vi "Read SecretKey.vi"(8 "error in (no error)":errorcluster, 11 "Attribute.Identity in":refnum<class "Attribute.Identity.lvclass">) -> (0 "error out":errorcluster, 2 "SecretKey":string, 3 "Attribute.Identity out":refnum<class "Attribute.Identity.lvclass">)   [LabVIEW 2013, in "Attribute.Identity.lvclass"]
uses:
  Attribute.Identity.lvclass
  Attribute.Identity.lvclass/Attribute.Identity.ctl
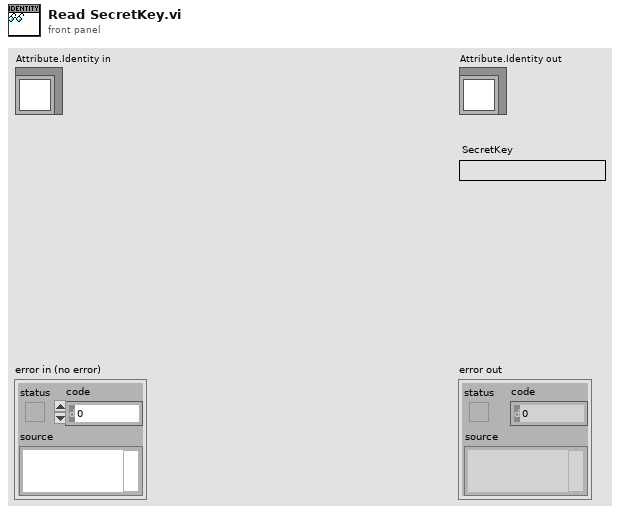
[diagram p1: front panel]
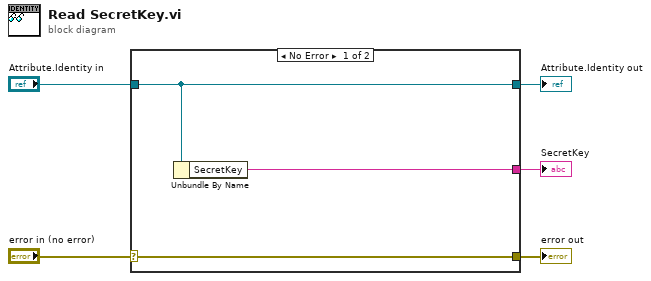
[diagram p0: block diagram]
diagram:
  n1 = case shown="No Error" "error in (no error)" {
    selector: "error in (no error)" -> [w8 w9]
    tunnel: [w8 w9] -> w4
    tunnel: [w7 w10] -> w2
    tunnel: "Attribute.Identity in" -> [w7 w10]
    tunnel: [w6 _] -> w1
    frame No Error {
      n2 = Unbundle By Name(w7) -> ("SecretKey"=w6:string)
    }
    frame Error {
    }
  }
  "error out" <- w4
  "Attribute.Identity out" <- w2
  "SecretKey" <- w1
